vi "SetPointToInteger.vi"(9 "RANGE":i32, 11 "SP OHMS":dbl) -> (3 "SP INTEGER":u16)   [LabVIEW 2021]
doc: "Converts temperature control set point,\ngiven in ohms, to an integer representation\nrequired by TS-530A."
panel:
  # "SetPointToInteger.vi"
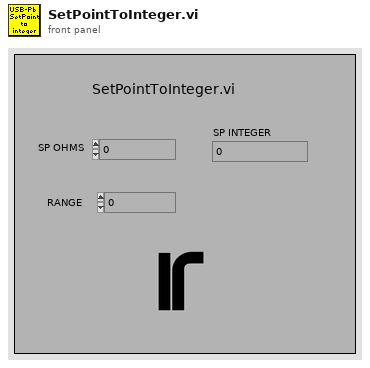
[diagram p1: front panel]
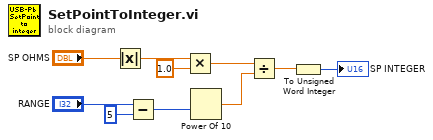
[diagram p0: block diagram]
diagram:
  n1 = Absolute Value(x="SP OHMS") -> (abs(x)=w3:dbl)
  n2 = Subtract(x="RANGE", y=u8 5) -> (x-y=w7:i32)
  n3 = Multiply(x=w3, y=1.0) -> (x*y=w10:dbl)
  n4 = Power Of 10(x=w7) -> (10^x=w9:dbl)
  n5 = Divide(x=w10, y=w9) -> (x/y=w2:dbl)
  n6 = To Unsigned Word Integer(number=w2) -> (unsigned 16bit integer=→"SP INTEGER":u16)
